vi "Module Not Synced--error.vi"() -> (0 "error out":errorcluster)   [LabVIEW 2025, in "Sequencer.lvlib"]
doc: "Outputs an error cluster containing a custom error code indicating the module events were unable to synchronize.\n_____\nBased on DQMH Dev Tools: Project Template 7.1.2.1547."
uses:
  Sequencer.lvlib
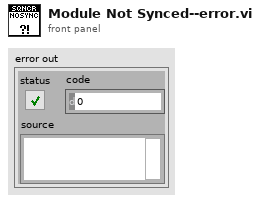
[diagram p1: front panel]
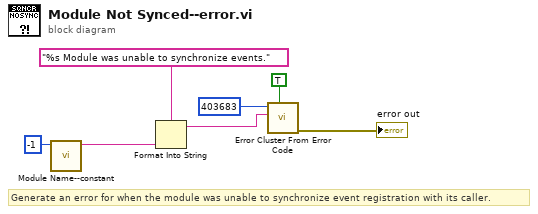
[diagram p0: block diagram]
diagram:
  # "Generate an error for when the module was unable to synchronize event registration with its caller."
  n1 = call "Module Name--constant.vi"("Module ID"=-1) -> ("Module Name"=w2:string)  [unwired: 10 in]
  n2 = Format Into String(format string="%s Module was unable to synchronize events.", w2) -> (resulting string=w6:string)  [unwired: 2 in, 1 out]
  n3 = call <vilib>:"Error Cluster From Error Code.vi"("show call chain? (False)"=TRUE, "error message (\"\")"=w6, "error code (0)"=403683) -> ("error out"=→"error out":errorcluster)  [unwired: 6 in]
